vi "Configure.vi"(8 "error in":errorcluster, 10 "name":string="CRDS", 11 "cCRDS in":refnum<class "cCRDS.lvclass">) -> (0 "error out":errorcluster, 3 "cCRDS out":refnum<class "cCRDS.lvclass">)   [LabVIEW 2012, in "cCRDS.lvclass"]
doc: "Configures the CRDS for operation and starts all DAQmx tasks associated with the instrument. This VI overrides the parent VI in the Instrument class."
uses:
  cCRDS.lvclass
  Cell/cCRDS Cell.lvclass
  Main Class/Controls/Get Tau Method.ctl
  Cell Class/CRDS Cell.lvclass
  Reusable/CRDS/Main/CRDS.lvclass
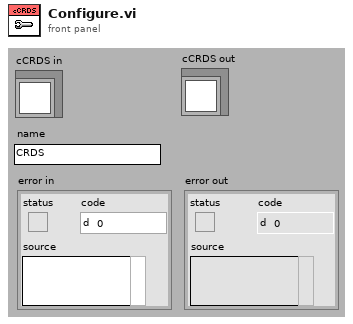
[diagram p1: front panel]
types:
  T1 = cluster{"Enable":refnum<k21>, "Clock":refnum<k21>}
  T2 = cluster{"Enable":refnum<k21>, "Setpoint":refnum<k21>}
  T3 = cluster{"HF AI":refnum<k21>, "LF AI":refnum<k21>}
  T4 = typedef "Get Tau Method.ctl" = enum8{"DFT-1", "DFT-5", "LRS"}
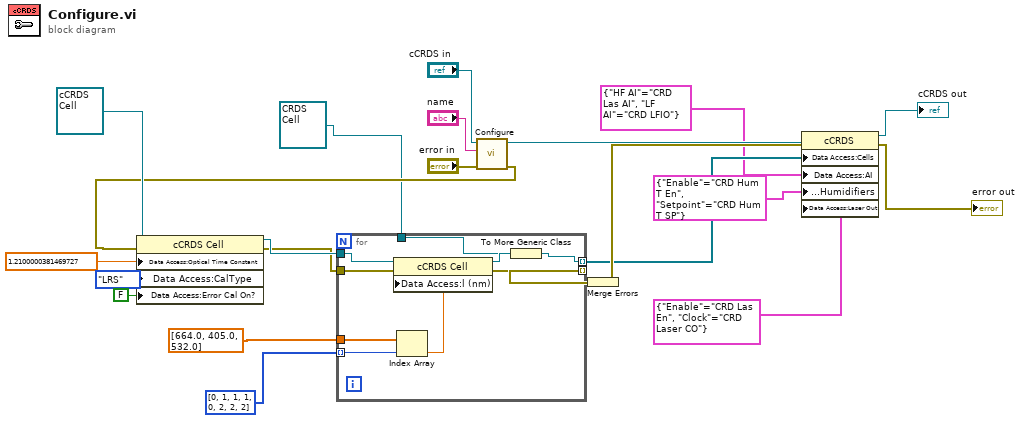
[diagram p0: block diagram]
diagram:
  n1 = call-parent "Configure.vi"("error in"="error in", "name"="name", "CRDS in"="cCRDS in") -> ("error out"=w9:errorcluster, "CRDS out"=w20:refnum<class "cCRDS.lvclass">)  [unwired: 7 in]
  n2 = property class="cCRDS Cell"(reference=refnum<class "cCRDS Cell.lvclass"> refnum ("cCRDS Cell"), error in=w9, "Data Access:Optical Time Constant"=sgl 1.21 ("Cavity Length (m)"), "Data Access:CalType"=Get_Tau_Method."LRS" ("CalType"), "Data Access:Error Cal On?"=FALSE ("Error Cal On?")) -> (reference out=w14:refnum<class "cCRDS Cell.lvclass">, error out=w8:errorcluster)
  n3 = for {
    tunnel: w14 -> [w29]
    tunnel: sgl[] [664.0, 405.0, 532.0] -> [w31]
    tunnel: i32[] [0, 1, 1, 1, 0, 2, 2, 2] -> [w30] mode=indexing
    tunnel: [w24] -> w4 mode=indexing
    tunnel: w8 -> [w27]
    tunnel: [w26] -> w7 mode=indexing
    tunnel: refnum<class "CRDS Cell.lvclass"> refnum ("CRDS Cell") -> [w23]
    n4 = Index Array(array=w31, index=w30) -> (element=w28:sgl)
    n5 = property class="cCRDS Cell"(reference=w29, error in=w27, "Data Access:l (nm)"=w28) -> (reference out=w25:refnum<class "cCRDS Cell.lvclass">, error out=w26:errorcluster)
    n6 = To More Generic Class(target class=w23, reference=w25) -> (generic class reference=w24:refnum<class "CRDS Cell.lvclass">)
  }
  n7 = Merge Errors(w7) -> (w6:errorcluster)
  n8 = property class="cCRDS"(reference=w20, error in=w6, "Data Access:Cells"=w4, "Data Access:AI"=T3 {"HF AI"="CRD Las AI", "LF AI"="CRD LFIO"} ("AI"), "Data Access:Humidifiers"=T2 {"Enable"="CRD Hum T En", "Setpoint"="CRD Hum T SP"} ("Humidifiers"), "Data Access:Laser Out"=T1 {"Enable"="CRD Las En", "Clock"="CRD Laser CO"} ("Laser Out")) -> (reference out=→"cCRDS out":refnum<class "cCRDS.lvclass">, error out=→"error out":errorcluster)
